vi "Task_LogFile.vi"(9 "Event Error":refnum<user-event>, 10 "File For Save":refnum<queue>, 11 "Class CSV_File":refnum<class "Class CSV_File.lvclass">) -> ()   [LabVIEW 2020, in "Library Instrument & Equipement.lvlib" / "Library Log_File.lvlib" / "Class Log_File Altyor.lvclass"]
uses:
  Class Log_File Altyor.lvclass
  Commun VI/TypeDef/Commande Test/Commande Data Test.ctl
  Commun VI/TypeDef/Commande Test/Commande Value Type.ctl
  Commun VI/TypeDef/Commande Test/Commande Type Test.ctl
  Read CSV File/CSV_File (Default)/Class CSV_File.lvclass
  C:/Users/ngarcin/OneDrive - Altyor/Standard TB/Suite TB45/Class/Read CSV File/Class File (Default)/Class File (Default).lvclass
  Commun VI/TypeDef/Variable Printable.ctl
  Commun VI/Library Commun.lvlib
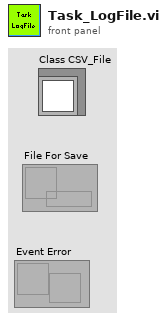
[diagram p1: front panel]
types:
  T1 = typedef "Library Commun.lvlib/Commande Data Test.ctl" = cluster{"Main Test":string, "Name Test":string, "StartOfTest":string, "Value":string, "Limit_Low":string, "Limit_High":string, "Result":bool, "Fatal_Test":bool, "NbRetry":dbl, "EndOfTest":string, "Error":string, "TypeValue":T2, "Type Test":T3}
  T2 = typedef "Library Commun.lvlib/Commande Value Type.ctl" = enum16{"None", "String", "Number", "Timestamp", "Boolean", "Array"}
  T3 = typedef "Library Commun.lvlib/Commande Type Test.ctl" = enum16{"Function", "Test", "Calculation"}
  T4 = typedef "Variable Printable.ctl" = string
  T5 = enum16{"Get Variable", "Get All Variables", "Set Variable", "Delete Variable", "Delete All Variable"}
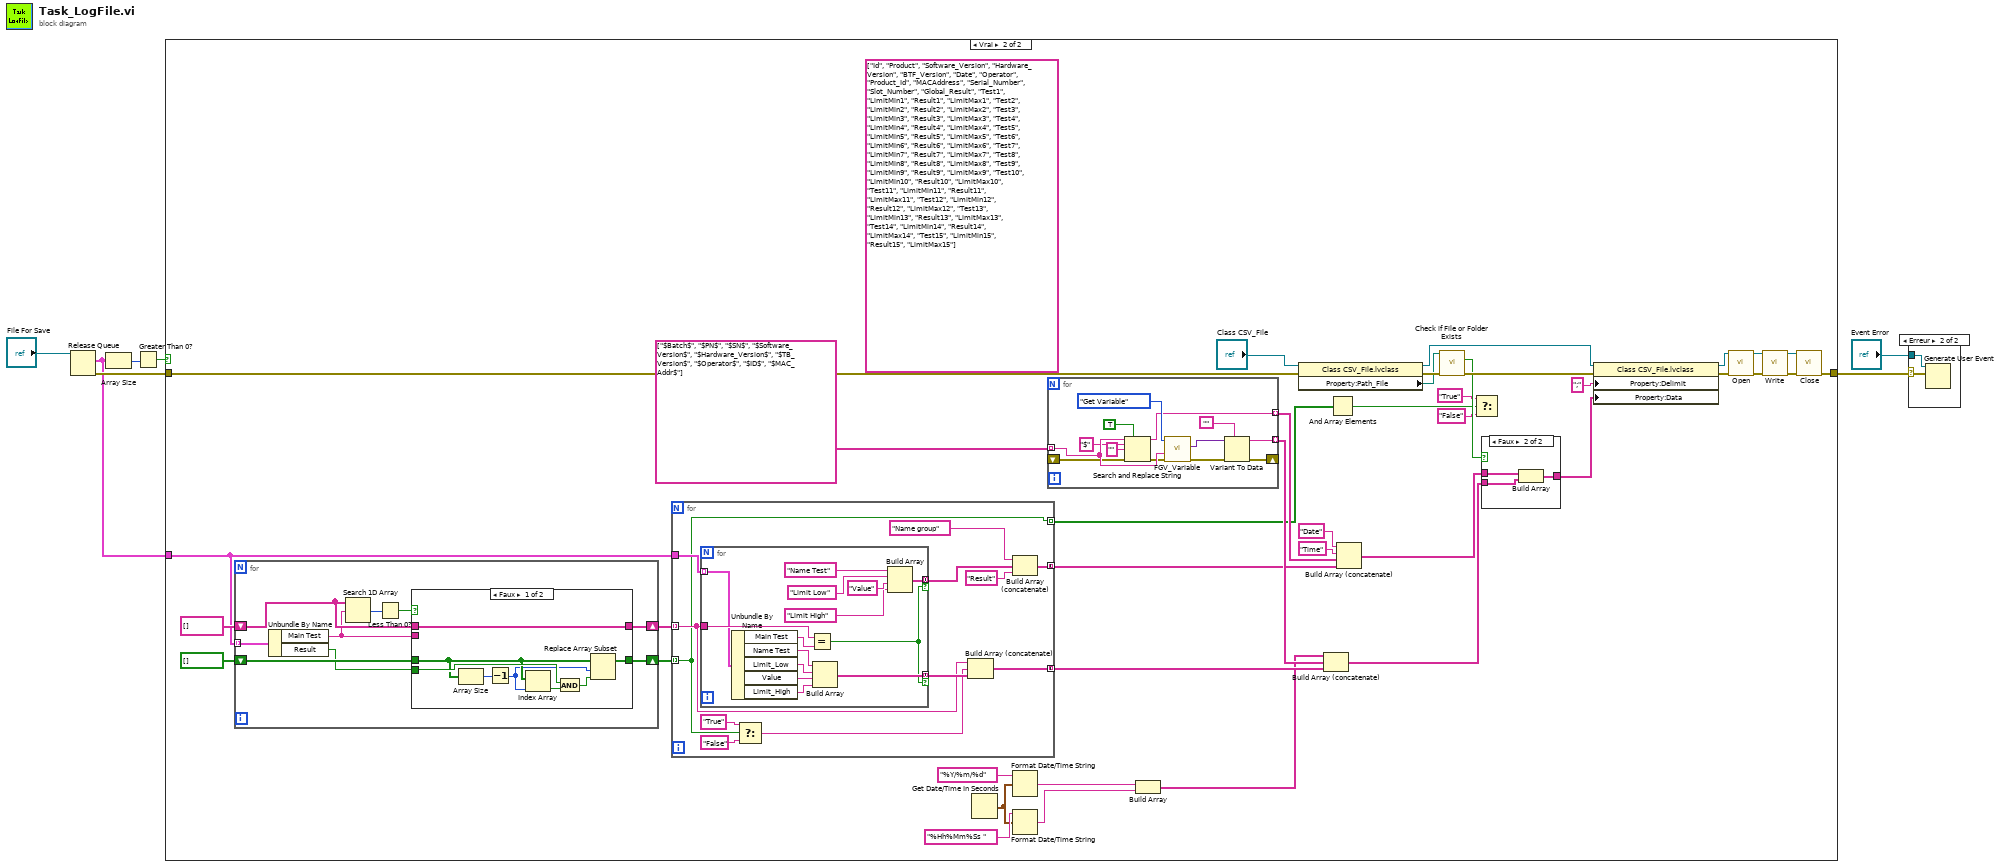
[diagram p0: block diagram]
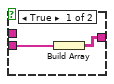
[diagram p3: hidden frame]
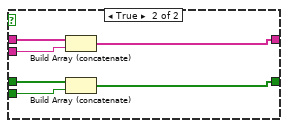
[diagram p4: hidden frame]
diagram:
  n1 = Release Queue(queue="File For Save") -> (remaining elements=w3:T1[], error out=w5:errorcluster)  [unwired: 2 in, 1 out]
  n2 = Array Size(array=w3) -> (size(s)=w2:i32)
  n3 = Greater Than 0?(x=w2) -> (x > 0?=w1:bool)
  n4 = case shown="Vrai" w1 {
    tunnel: [w8 w36] -> w6
    tunnel: w5 -> [w8 w23]
    tunnel: w3 -> [_ w42]
    frame False {
    }
    frame True {
      (unwired) string[] ["Id", "Product", "Software_Version", "Hardware_Version", "BTF_Version", "Date", "Operator", "Product_Id", "MACAddress", "Serial_Number", "Slot_Number", "Global_Result", "Test1", "LimitMin1", "Result1", "LimitMax1", "Test2", "LimitMin2", "Result2", "LimitMax2", "Test3", "LimitMin3", "Result3", "LimitMax3", "Test4", "LimitMin4", "Result4", "LimitMax4", "Test5", "LimitMin5", "Result5", "LimitMax5", "Test6", "LimitMin6", "Result6", "LimitMax6", "Test7", "LimitMin7", "Result7", "LimitMax7", "Test8", "LimitMin8", "Result8", "LimitMax8", "Test9", "LimitMin9", "Result9", "LimitMax9", "Test10", "LimitMin10", "Result10", "LimitMax10", "Test11", "LimitMin11", "Result11", "LimitMax11", "Test12", "LimitMin12", "Result12", "LimitMax12", "Test13", "LimitMin13", "Result13", "LimitMax13", "Test14", "LimitMin14", "Result14", "LimitMax14", "Test15", "LimitMin15", "Result15", "LimitMax15"] ("Columns")
      n5 = for {
        tunnel: w42 -> [w88] mode=indexing
        shift-right: [w83] -> w46
        shift-left: string[] [] -> [w85]
        shift-right: [w80] -> w43
        shift-left: bool[] [] -> [w82]
        n6 = Unbundle By Name(w88) -> ("Main Test"=w84:string, "Result"=w81:bool)
        n7 = Search 1D Array(1D array=w85, element=w84) -> (index of element=w87:i32)  [unwired: 1 in]
        n8 = Less Than 0?(x=w87) -> (x < 0?=w86:bool)
        n9 = case shown="Faux" w86 {
          tunnel: w85 -> [w96 w102]
          tunnel: w84 -> [_ w101]
          tunnel: [w96 w100] -> w83
          tunnel: w82 -> [w92 w99]
          tunnel: w81 -> [w94 w98]
          tunnel: [w89 w97] -> w80
          frame False {
            n10 = Array Size(array=w92) -> (size(s)=w95:i32)
            n11 = Decrement(x=w95) -> (x-1=w91:i32)
            n12 = Index Array(array=w92, index=w91) -> (element=w93:bool)
            n13 = And(x=w94, y=w93) -> (x .and. y?=w90:bool)
            n14 = Replace Array Subset(array=w92, new element=w90, index=w91) -> (w89:bool[])
          }
          frame True {
            n15 = Build Array (concatenate)(w102, w101) -> (w100:string[])
            n16 = Build Array (concatenate)(w99, w98) -> (w97:bool[])
          }
        }
      }
      n17 = for {
        tunnel: w46 -> [w61] mode=indexing
        tunnel: w42 -> [w65]
        tunnel: w43 -> [w54] mode=indexing
        tunnel: [w59] -> w44 mode=concatenating
        tunnel: [w55] -> w26 mode=concatenating
        tunnel: [w54] -> w11 mode=indexing
        n18 = for {
          tunnel: w65 -> [w78] mode=indexing
          tunnel: w61 -> [w79]
          tunnel: [w74] -> w62 mode=concatenating if=w66
          tunnel: [w67] -> w57 mode=concatenating if=w66
          n19 = Unbundle By Name(w78) -> ("Main Test"=w72:string, "Name Test"=w73:string, "Limit_Low"=w77:string, "Value"=w76:string, "Limit_High"=w75:string)
          n20 = Equal?(x=w79, y=w72) -> (x = y?=w66:bool)
          n21 = Build Array(w73, w77, w76, w75) -> (w74:string[])
          n22 = Build Array("Name Test", "Limit Low" ("élément"), "Value" ("élément"), "Limit High" ("élément")) -> (w67:string[])
        }
        n23 = Select(t="True", s=w54, f="False") -> (s? t:f=w60:string)
        n24 = Build Array (concatenate)(w61, w60, w62) -> (w59:string[])
        n25 = Build Array (concatenate)("Name group", w57, "Result" ("élément")) -> (w55:string[])
      }
      n26 = Get Date/Time In Seconds() -> (seconds since 1Jan1904=w31:timestamp)
      n27 = Format Date/Time String(time format string (%c)="%Y/%m/%d" ("chaîne de format de l'heure (%c)"), seconds (now)=w31) -> (date/time string=w30:string)  [unwired: 1 in]
      n28 = Format Date/Time String(time format string (%c)="%Hh%Mm%Ss " ("chaîne de format de l'heure (%c)"), seconds (now)=w31) -> (date/time string=w29:string)  [unwired: 1 in]
      n29 = for {
        tunnel: [w112] -> w34 mode=indexing
        shift-right: [w110] -> _
        shift-left: _ -> [w108]
        tunnel: T4[] ["$Batch$", "$PN$", "$SN$", "$Software_Version$", "$Hardware_Version$", "$TB_Version$", "$Operator$", "$ID$", "$MAC_Addr$"] ("Columns") -> [w109] mode=indexing
        tunnel: [w104] -> w27 mode=indexing
        n30 = Search and Replace String(replace all?=TRUE ("tout remplacer ? (F)"), input string=w109, search string="$" ("chaîne recherchée"), replace string="" ("chaîne de remplacement (\"\")"), error in=w108) -> (result string=w104:string, error out=w107:errorcluster)  [unwired: 3 in, 2 out]
        n31 = call "FGV_Variable.vi"("error in (no error)"=w107, "Variable"=w109, "Function"=T5."Get Variable") -> ("error out"=w111:errorcluster, "Data Out"=w114:variant)  [unwired: 6 in, 1 out]
        n32 = Variant To Data(error in=w111, type="", Variant=w114) -> (data=w112:string, error out=w110:errorcluster)
      }
      n33 = Build Array(w30, w29) -> (w28:string[])
      n34 = property class="Class CSV_File.lvclass"(reference="Class CSV_File", error in=w23) -> (reference out=w21:refnum<class "Class CSV_File.lvclass">, error out=w20:errorcluster, "Property:Path_File"=w18:path)
      n35 = Build Array (concatenate)(w28, w34, w44) -> (w17:string[])
      n36 = And Array Elements(Boolean array=w11) -> (logical AND=w10:bool)
      n37 = Build Array (concatenate)("Date" ("chaîne recherchée"), "Time" ("chaîne recherchée"), w27, w26) -> (w14:string[])
      n38 = call <vilib>:"Check if File or Folder Exists.vi"("error in (no error)"=w20, "path"=w18) -> ("error out"=w19:errorcluster, "file or folder exists?"=w15:bool)  [unwired: 7 in, 1 out]
      n39 = Select(t="True", s=w10, f="False") -> ()  [unwired: 1 out]
      n40 = case shown="Faux" w15 {
        tunnel: w17 -> [w50 w53]
        tunnel: [w49 w52] -> w16
        tunnel: w14 -> [_ w51]
        frame True {
          n41 = Build Array(w50) -> (w49:string[][])
        }
        frame False {
          n42 = Build Array(w51, w53) -> (w52:string[][])
        }
      }
      n43 = property class="Class CSV_File.lvclass"(reference=w21, error in=w19, "Property:Delimit"=";" ("Delimit"), "Property:Data"=w16) -> (reference out=w41:refnum<class "Class CSV_File.lvclass">, error out=w39:errorcluster)
      n44 = call-dynamic "Open.vi"("error in (no error)"=w39, "Class CSV_File (Default) en entrée"=w41) -> ("error out"=w38:errorcluster, "Class CSV_File (Default) en sortie"=w40:refnum<class "Class CSV_File.lvclass">)  [unwired: 8 in]
      n45 = call-dynamic "Write.vi"("error in (no error)"=w38, "Class CSV_File (Default) en entrée"=w40) -> ("error out"=w37:errorcluster, "Class CSV_File (Default) en sortie"=w35:refnum<class "Class CSV_File.lvclass">)  [unwired: 8 in]
      n46 = call-dynamic "Close.vi"("error in (no error)"=w37, "Class CSV_File (Default) en entrée"=w35) -> ("error out"=w36:errorcluster)  [unwired: 8 in, 1 out]
    }
  }
  n47 = case shown="Erreur" w6 {
    selector: w6 -> [_ w116]
    tunnel: "Event Error" -> [_ w117]
    frame No Error {
    }
    frame Error {
      n48 = Generate User Event(user event=w117, event data cluster=w116) -> ()  [unwired: 2 in, 2 out]
    }
  }
